vi "P3060_DMA写U64数据.vi"(6 "写U8数据":u64[](array[numeric]), 8 "错误输入":errorcluster caption="错误输入（无错误）", 10 "偏移地址":u32, 11 "句柄输入":i32) -> (0 "错误输出":errorcluster, 2 "返回值":i32, 3 "句柄输出":i32)   [LabVIEW 2010]
doc: "发送异步通道数据"
uses:
  dll/P3060.dll
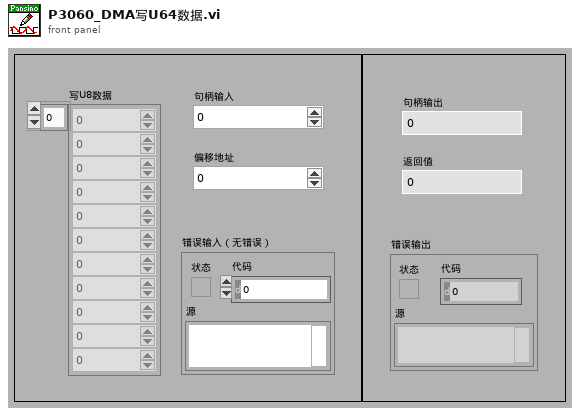
[diagram p1: front panel]
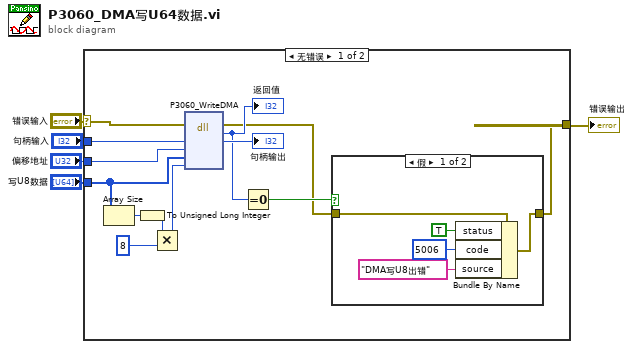
[diagram p0: block diagram]
diagram:
  n1 = case shown="无错误" "错误输入" {
    selector: "错误输入" -> [w18 w25]
    tunnel: [w12 w25] -> w4
    tunnel: "句柄输入" -> [w16 _]
    tunnel: "写U8数据" -> [w6 _]
    tunnel: "偏移地址" -> [w11 _]
    frame No Error {
      n2 = Array Size(array=w6) -> (size(s)=w8:i32)
      n3 = To Unsigned Long Integer(number=w8) -> (unsigned 32bit integer=w9:u32)
      n4 = Multiply(x=w9, y=u32 8) -> (x*y=w7:u32)
      n5 = dll-call lib="D:/driver/trunk/Drivers/P3060/P3060API/P3060APILV/Labview/P3060/_SubVI/dll/P3060.dll" fn="P3060_WriteDMA"(error in=w18, "hDev"=w16, "Offset"=w11, "pBuffer"=w6, "lengthToWrite"=w7) -> (error out=w13:errorcluster, "return"=w15:i32, "hDev"=→"句柄输出":i32)  [unwired: 5 in, 1 out]
      "返回值" <- w15
      n6 = Equal To 0?(x=w15) -> (x = 0?=w14:bool)
      n7 = case shown="假" w14 {
        tunnel: [w22 w24] -> w12
        tunnel: w13 -> [w23 w24]
        frame False {
          n8 = Bundle By Name(cluster=w23, "status"=TRUE, "code"=5006, "source"="DMA写U8出错") -> (w22:errorcluster)
        }
        frame True {
        }
      }
    }
    frame Error {
    }
  }
  "错误输出" <- w4
